vi "SHA-1.vi"(8 "error in (no error)":errorcluster, 11 "Message":u8[](array[numeric]) format="%.0x") -> (0 "error out":errorcluster, 1 "ASCII Formatted hash":string, 3 "Hash":u8[](array[numeric]))   [LabVIEW 2011, in "i3-external-encryption.lvlib"]
uses:
  i3-external-encryption.lvlib
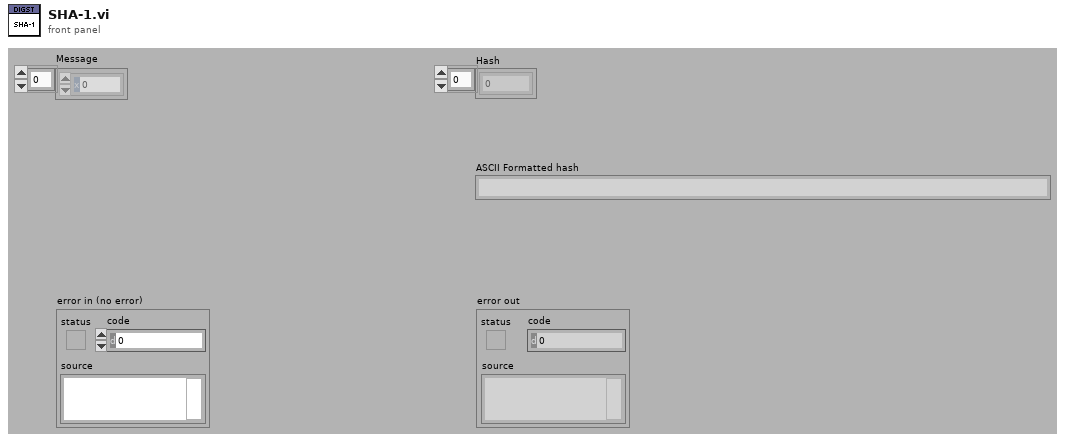
[diagram p1: front panel]
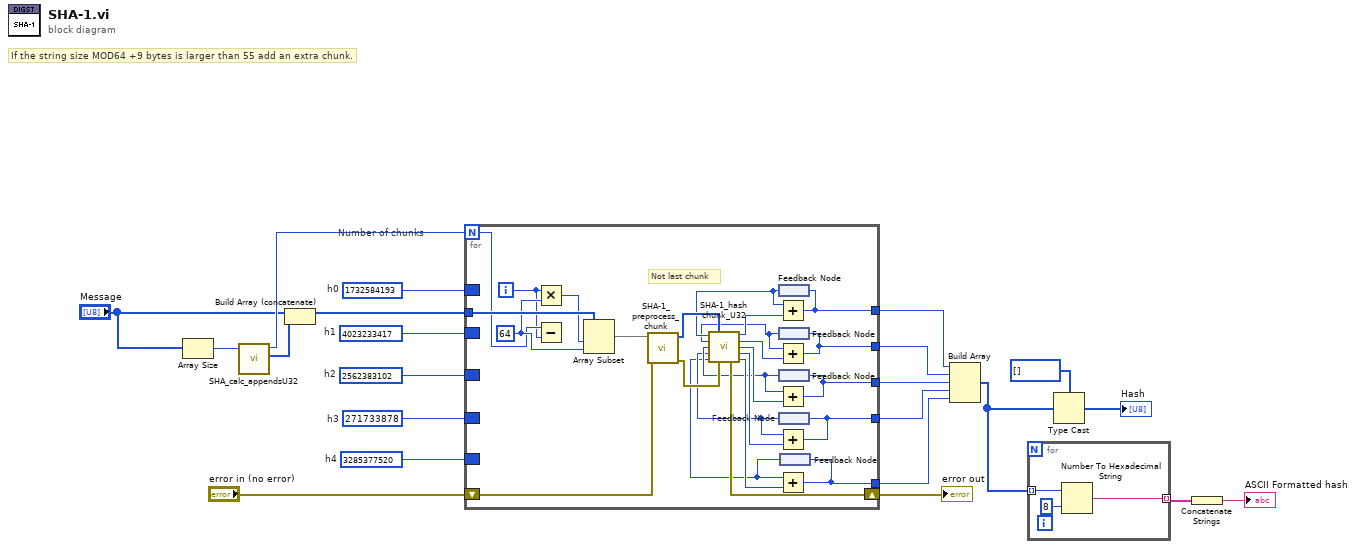
[diagram p0: block diagram]
diagram:
  w13 = u32 3285377520  # h4
  w14 = u32 271733878  # h3
  w15 = u32 2562383102  # h2
  w16 = u32 4023233417  # h1
  w17 = u32 1732584193  # h0
  # "Number of chunks"
  # "If the string size MOD64 +9 bytes is larger than 55 add an extra chunk."
  n1 = Array Size(array="Message") -> (size(s)=w11:i32)
  n2 = call "SHA_calc_appendsU32.vi"("String length"=w11) -> ("Append"=w6:u8[], "Number of chunks"=w12:i32)  [unwired: 9 in]
  n3 = Build Array (concatenate)("Message", w6) -> (w4:u8[])
  n4 = for {
    N: w12 -> [w44]
    tunnel: w4 -> [w47]
    tunnel: [w41] -> w22
    tunnel: [w40] -> w21
    tunnel: [w39] -> w20
    tunnel: [w38] -> w19
    tunnel: [w42] -> w18
    border: w13 -> [_]
    border: w17 -> [_]
    border: w16 -> [_]
    border: w15 -> [_]
    border: w14 -> [_]
    shift-right: [w32] -> w10
    shift-left: "error in (no error)" -> [w31]
    i -> [w43]
    w45 = 64 ("x")
    # "Not last chunk"
    n5 = Multiply(x=w43, y=w45) -> (x*y=w46:i32)
    n6 = Subtract(x=w44, y=w43) -> ()  [unwired: 1 out]
    n7 = Array Subset(array=w47, index=w46, length=w45) -> (w23:u8[])
    n8 = call "SHA-1_preprocess_chunk.vi"("error in (no error)"=w31, "Chunk in"=w23) -> ("error out"=w29:errorcluster, "Processed chunk out"=w30:u32[])  [unwired: 8 in]
    n9 = feedback #1() -> (w28:u32)
    n10 = feedback #2() -> (w27:u32)
    n11 = feedback #3() -> (w26:u32)
    n12 = feedback #4() -> (w25:u32)
    n13 = feedback #5() -> (w24:u32)
    n14 = call "SHA-1_hash chunk_U32.vi"("h0"=w28, "Chunk"=w30, "h1"=w27, "h2"=w26, "h3"=w25, "h4"=w24, "error in (no error)"=w29) -> ("a"=w37:u32, "b"=w36:u32, "c"=w35:u32, "d"=w34:u32, "error out"=w32:errorcluster, "e"=w33:u32)  [unwired: 3 in]
    n15 = Add(x=w28, y=w37) -> (x+y=w41:u32)
    n16 = Add(x=w27, y=w36) -> (x+y=w40:u32)
    n17 = Add(x=w26, y=w35) -> (x+y=w39:u32)
    n18 = Add(x=w25, y=w34) -> (x+y=w38:u32)
    n19 = Add(x=w24, y=w33) -> (x+y=w42:u32)
    n20 = feedback-in #1(w41) -> ()
    n21 = feedback-in #2(w40) -> ()
    n22 = feedback-in #3(w39) -> ()
    n23 = feedback-in #4(w38) -> ()
    n24 = feedback-in #5(w42) -> ()
  }
  "error out" <- w10
  n25 = Build Array(w22, w21, w20, w19, w18) -> (w3:u32[])
  n26 = for {
    tunnel: w3 -> [w50] mode=indexing
    tunnel: [w48] -> w8 mode=indexing
    n27 = Number To Hexadecimal String(1:i16 8 ("width (-)"), 2:w50) -> (0:w48:string)
  }
  n28 = Type Cast(type=u8[] [] ("Hash"), x=w3) -> (*(type *) &x=→"Hash":u8[])
  n29 = Concatenate Strings(w8) -> (→"ASCII Formatted hash":string)
